vi "RandomValuesSelectionV2.2.vi"(3 "Number of Columns":i32, 4 "Number of  Rows":i32, 6 "Number of Mine":i32) -> (1 "FullMap":i32[][](array[numeric]), 2 "FirstClikPosition":i32[](array[numeric]))   [LabVIEW 2014]
panel:
  out "AllZero":i32[][](array[numeric])
  out "MineAround":i32
  out "FirstNum":i32
  out "OnlyMine":i32[][](array[numeric])
  out "Ramdom Array":i32[](array[numeric])
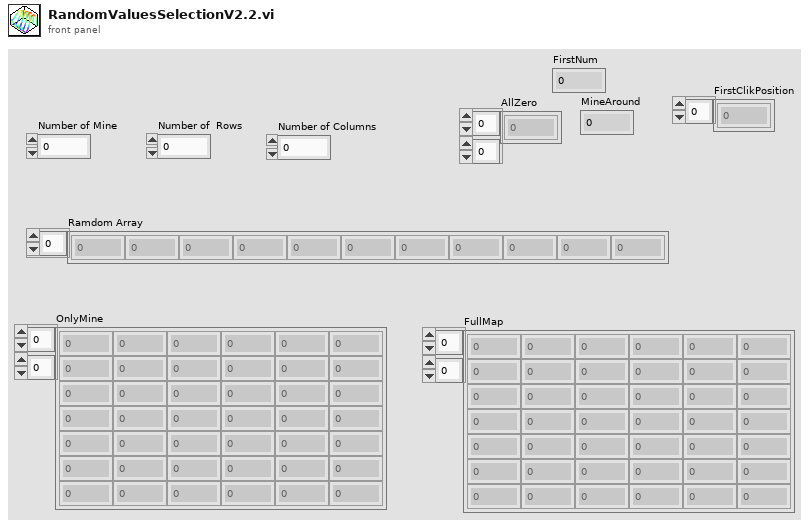
[diagram p1: front panel]
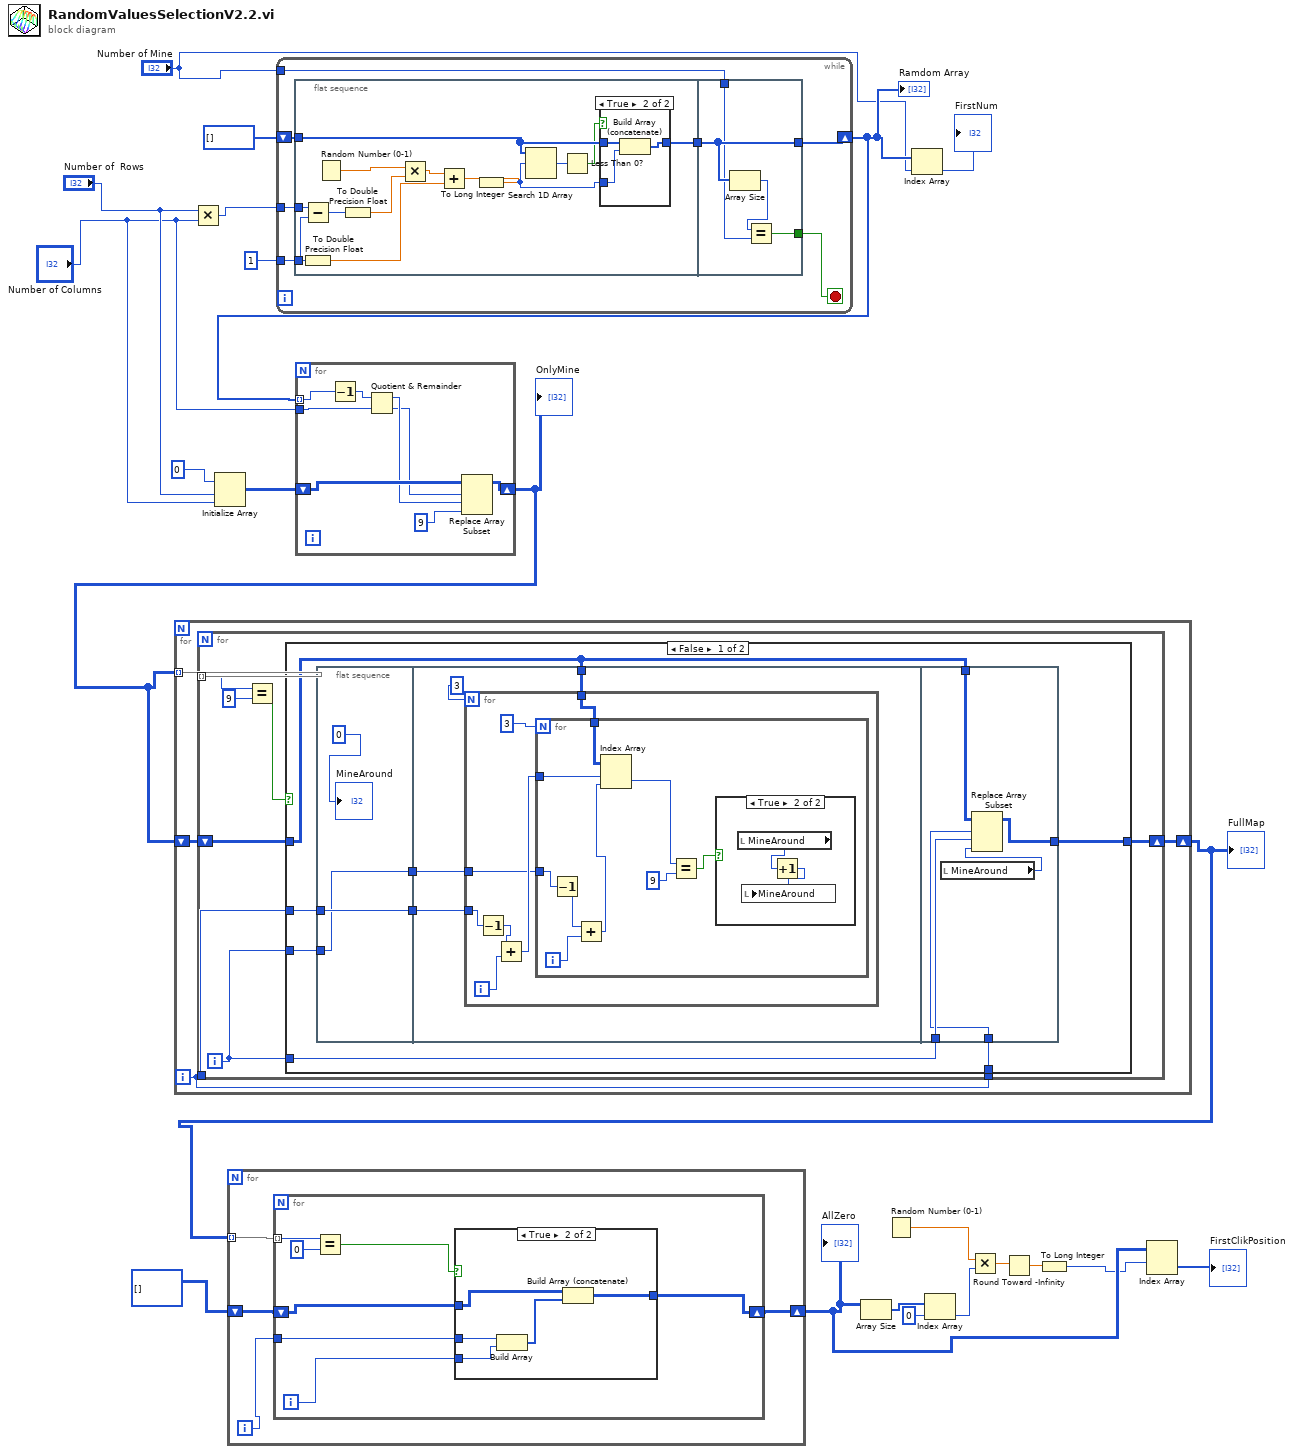
[diagram p0: block diagram]
diagram:
  n1 = Multiply(x="Number of  Rows", y="Number of Columns") -> (x*y=w20:i32)
  n2 = Initialize Array(0 ("element"), "Number of  Rows", "Number of Columns") -> (w17:i32[][])
  n3 = while {
    tunnel: 1 ("1") -> [w29]
    shift-right: [w28] -> w16
    shift-left: i32[] [] -> [w27]
    tunnel: w20 -> [w26]
    tunnel: "Number of Mine" -> [w24]
    stop <- w23 stop-if-true
    n4 = flat-sequence {
      tunnel: w29 -> [w41]
      tunnel: w27 -> [w34]
      tunnel: w26 -> [w30]
      tunnel: [w35] -> w25
      tunnel: [w50] -> w28
      tunnel: w25 -> [w50]
      tunnel: w24 -> [w48]
      tunnel: [w47] -> w23
      frame #0 {
        n5 = Subtract(x=w30, y=w41) -> (x-y=w42:i32)
        n6 = To Double Precision Float(number=w41) -> (double precision float=w40:dbl)
        n7 = Random Number (0-1)() -> (number: 0 to 1=w38:dbl)
        n8 = To Double Precision Float(number=w42) -> (double precision float=w37:dbl)
        n9 = Multiply(x=w38, y=w37) -> (x*y=w36:dbl)
        n10 = Add(x=w36, y=w40) -> (x+y=w39:dbl)
        n11 = To Long Integer(number=w39) -> (32bit integer=w33:i32)
        n12 = Search 1D Array(1D array=w34, element=w33) -> (index of element=w31:i32)  [unwired: 1 in]
        n13 = Less Than 0?(x=w31) -> (x < 0?=w32:bool)
        n14 = case shown="True" w32 {
          tunnel: w33 -> [_ w46]
          tunnel: [w43 w45] -> w35
          tunnel: w34 -> [w43 w44]
          frame False {
          }
          frame True {
            n15 = Build Array (concatenate)(w44, w46) -> (w45:i32[])
          }
        }
      }
      frame #1 {
        n16 = Array Size(array=w50) -> (size(s)=w49:i32)
        n17 = Equal?(x=w49, y=w48) -> (x = y?=w47:bool)
      }
    }
  }
  "Ramdom Array" <- w16
  n18 = for {
    tunnel: w16 -> [w57] mode=indexing
    tunnel: "Number of Columns" -> [w58]
    shift-right: [w51] -> w13
    shift-left: w17 -> [w55]
    n19 = Decrement(x=w57) -> (x-1=w56:i32)
    n20 = Quotient & Remainder(x=w56, y=w58) -> (x-y*floor(x/y)=w54:i32, floor(x/y)=w53:i32)
    n21 = Replace Array Subset(array=w55, new element=9, index (row)=w53, index (col)=w54) -> (w51:i32[][])
  }
  "OnlyMine" <- w13
  n22 = for {
    tunnel: w13 -> [w62] mode=indexing
    shift-right: [w60] -> w11
    shift-left: w13 -> [w61]
    i -> [w59]
    n23 = for {
      tunnel: w62 -> [w70] mode=indexing
      tunnel: w59 -> [w65]
      tunnel: w59 -> [w63]
      shift-right: [w66] -> w60
      shift-left: w61 -> [w67]
      i -> [w64]
      n24 = Equal?(x=w70, y=9) -> (x = y?=w68:bool)
      n25 = case shown="False" w68 {
        tunnel: w67 -> [w74 w109]
        tunnel: [w71 w109] -> w66
        tunnel: w65 -> [w78 _]
        tunnel: w64 -> [w76 _]
        tunnel: w64 -> [w73 _]
        tunnel: w63 -> [w72 _]
        frame False {
          n26 = flat-sequence {
            tunnel: w78 -> [w80]
            tunnel: [w80] -> w77
            tunnel: w76 -> [w79]
            tunnel: [w79] -> w75
            tunnel: w74 -> [w84]
            tunnel: w77 -> [w83]
            tunnel: w75 -> [w82]
            tunnel: w74 -> [w108]
            tunnel: w73 -> [w107]
            tunnel: w72 -> [w106]
            tunnel: [w104] -> w71
            frame #0 {
              "MineAround" <- 0
            }
            frame #1 {
              n27 = for {
                N: 3 -> [_]
                tunnel: w84 -> [w91]
                tunnel: w83 -> [w90]
                tunnel: w82 -> [w86]
                i -> [w88]
                n28 = Decrement(x=w90) -> (x-1=w89:i32)
                n29 = Add(x=w89, y=w88) -> (x+y=w87:i32)
                n30 = for {
                  N: 3 -> [_]
                  tunnel: w91 -> [w100]
                  tunnel: w87 -> [w99]
                  tunnel: w86 -> [w98]
                  i -> [w97]
                  n31 = Decrement(x=w98) -> (x-1=w96:i32)
                  n32 = Add(x=w96, y=w97) -> (x+y=w95:i32)
                  n33 = Index Array(array=w100, index (row)=w99, index (col)=w95) -> (element=w94:i32)
                  n34 = Equal?(x=w94, y=9) -> (x = y?=w93:bool)
                  n35 = case shown="True" w93 {
                    frame False {
                    }
                    frame True {
                      n36 = local read "MineAround"() -> (w103:i32)
                      n37 = Increment(x=w103) -> (x+1=w102:i32)
                      n38 = local write "MineAround"(w102) -> ()
                    }
                  }
                }
              }
            }
            frame #2 {
              n39 = local read "MineAround"() -> (w105:i32)
              n40 = Replace Array Subset(array=w108, new element=w105, index (row)=w106, index (col)=w107) -> (w104:i32[][])
            }
          }
        }
        frame True {
        }
      }
    }
  }
  "FullMap" <- w11
  n41 = for {
    tunnel: w11 -> [w113] mode=indexing
    shift-right: [w110] -> w3
    shift-left: i32[][] [] -> [w112]
    i -> [w111]
    n42 = for {
      tunnel: w113 -> [w120] mode=indexing
      shift-right: [w114] -> w110
      shift-left: w112 -> [w117]
      tunnel: w111 -> [w116]
      i -> [w115]
      n43 = Equal?(x=w120, y=0) -> (x = y?=w118:bool)
      n44 = case shown="True" w118 {
        tunnel: w117 -> [w121 w124]
        tunnel: w116 -> [_ w126]
        tunnel: w115 -> [_ w125]
        tunnel: [w121 w122] -> w114
        frame False {
        }
        frame True {
          n45 = Build Array(w126, w125) -> (w123:i32[])
          n46 = Build Array (concatenate)(w124, w123) -> (w122:i32[][])
        }
      }
    }
  }
  "AllZero" <- w3
  n47 = Array Size(array=w3) -> (size(s)=w9:i32[])
  n48 = Random Number (0-1)() -> (number: 0 to 1=w7:dbl)
  n49 = Index Array(array=w16, index="Number of Mine") -> (element=→"FirstNum":i32)
  n50 = Index Array(array=w9, index=0) -> (element=w6:i32)
  n51 = Multiply(x=w7, y=w6) -> (x*y=w5:dbl)
  n52 = Round Toward -Infinity(1:w5) -> (0:w4:dbl)
  n53 = To Long Integer(number=w4) -> (32bit integer=w2:i32)
  n54 = Index Array(array=w3, index (row)=w2) -> (element=→"FirstClikPosition":i32[])  [unwired: 1 in]
